vi "_Read XIC.vi"(0 "file path":path, 7 "Expt#":i32=1, 9 "MR#":i32=1, 11 "error in (no error)":errorcluster) -> (4 "Data":T6, 6 "Expt# Out":i32=1, 8 "MR# Out":i32=1, 10 "Version":i32, 15 "error out":errorcluster)   [LabVIEW 2012]
uses:
  Type/_Data.ctl
  Type/_XML Expt.ctl
  Type/_XML Lens.ctl
  Type/_Mass Range Property.ctl
  Type/_Mass Range Parameters.ctl
  Type/_RT Res Type.ctl
  Type/_GUI Method.ctl
  Type/_Lens Property.ctl
  Type/_Run Mode.ctl
panel:
  out "Steps":i32[][](array[numeric])
  in  "AcqMethod":T1[](array[typedef]) {"ScanType" format="%#.6g"; "Mass Range"."Res" items=["High/High", "Medium/Medium", "Low/Low", "High/Medium", "High/Low", "Medium/High", "Medium/Low", "Low/High", "Low/Medium"]}
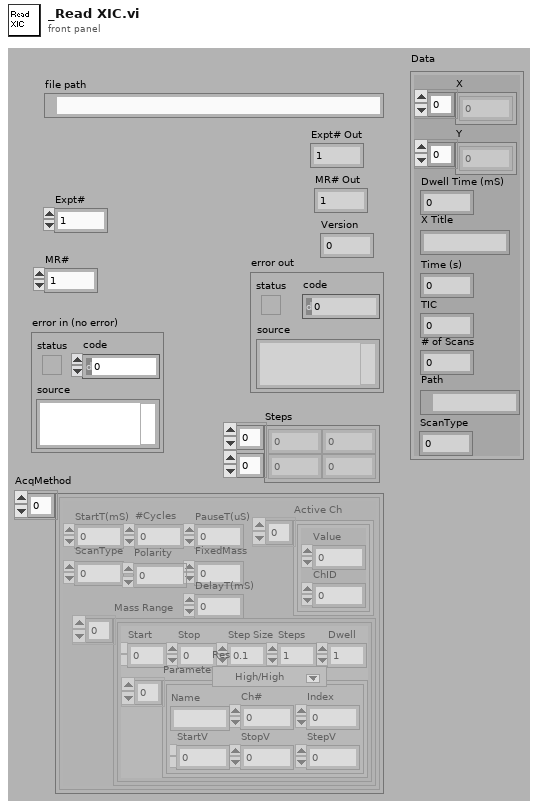
[diagram p1: front panel]
types:
  T1 = typedef "_XML Expt.ctl" = cluster{"StartT(mS)":i32, "#Cycles":i32, "PauseT(uS)":i32, "ScanType":i32, "Polarity":u8, "FixedMass":dbl, "DelayT(mS)":i32, "Active Ch":T2[], "Mass Range":T3[]}
  T2 = typedef "_XML Lens.ctl" = cluster{"Value":dbl, "ChID":u8}
  T3 = typedef "_Mass Range Property.ctl" = cluster{"Start":dbl, "Stop":dbl, "Step Size":dbl, "Steps":i32, "Dwell":dbl, "Parameters":T4[], "Res":T5}
  T4 = typedef "_Mass Range Parameters.ctl" = cluster{"Name":string, "Ch#":u8, "StartV":dbl, "StopV":dbl, "StepV":dbl, "Index":u8}
  T5 = typedef "_RT Res Type.ctl" = u16
  T6 = typedef "_Data.ctl" = cluster{"X":dbl[], "Y":dbl[], "Dwell Time (mS)":dbl, "X Title":string, "Time (s)":dbl, "TIC":u32, "# of Scans":i32, "Path":path, "ScanType":i32}
  T7 = typedef "_GUI Method.ctl" = cluster{"Lenses":T8[], "Mass Ranges":T3[], "Acquire":bool, "MCA":bool, "Q1DC EN":bool, "Q1 POL":bool, "Q3 POL":bool, "Q1 RF  EN":bool, "Averaging":bool, "Log Scale":bool, "CPS":bool, "Unit":bool, "Data Path":path, "Run Mode":T9, "Fixed Mass (amu)":dbl, "Q3DC EN":bool, "Q3 RF  EN":bool, "Negative":bool}
  T8 = typedef "_Lens Property.ctl" = cluster{"Scan Type":u8, "Scans":i32, "Time 1":dbl, "Time 2":dbl, "Value 1":dbl, "Value 2":dbl, "Step Size":dbl}
  T9 = typedef "_Run Mode.ctl" = enum16{"MRM (Q1/Q2)", "Q1 Scan", "Q1 SRM", "Q2 Scan", "Q2 SRM", "Product Scan", "Precursor Scan", "Neutral Loss", "Neutral Gain"}
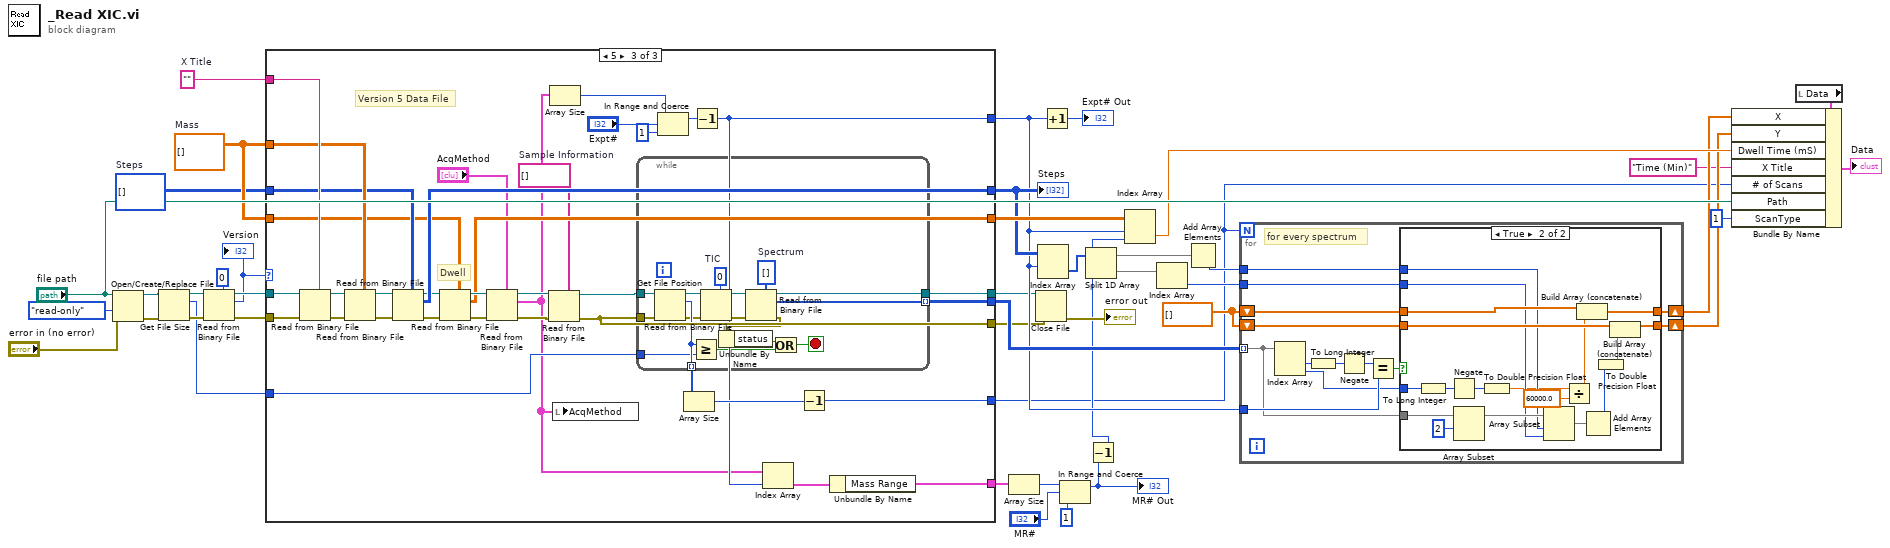
[diagram p0: block diagram]
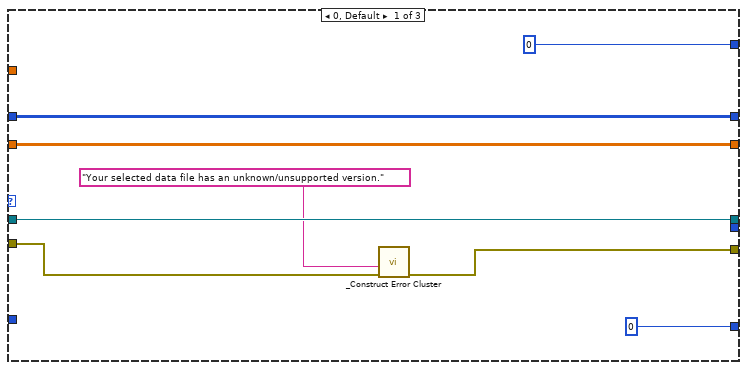
[diagram p3: hidden frame]
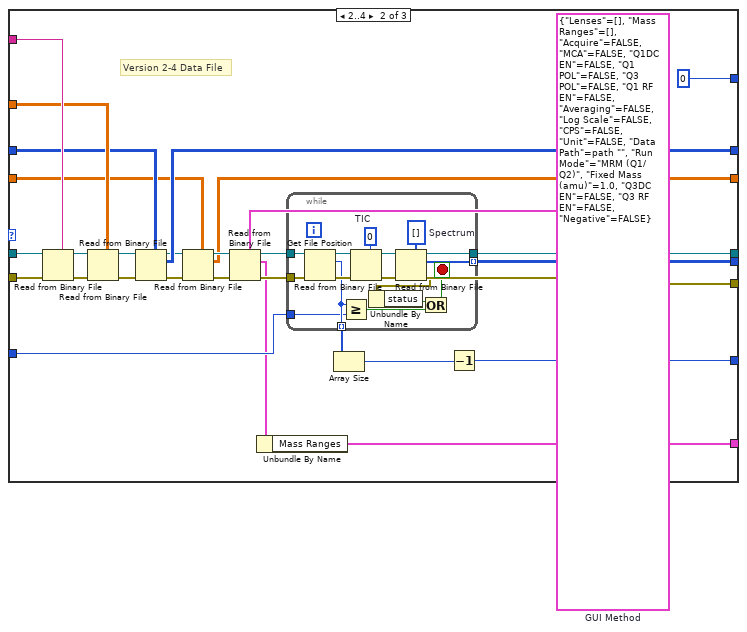
[diagram p4: hidden frame]
diagram:
  w11 = dbl[] [] ("subarray")
  w25 = ""  # X Title
  w26 = i32[][] []  # Steps
  w27 = dbl[][] []  # Mass
  n1 = Open/Create/Replace File(file path (use dialog)="file path", error in="error in (no error)", access (0:read/write)=enum16{"read/write", "read-only", "write-only"}."read-only") -> (refnum out=w38:refnum<file>, error out=w37:errorcluster)  [unwired: 4 out]
  n2 = Get File Size ("EOF")(file=w38, error in=w37) -> (refnum out=w34:refnum<file>, size (in bytes)=w30:i64, 0:w33:errorcluster)
  n3 = Read from Binary File(5:0 ("pos offset (0)"), 8:w33, 11:w34) -> (0:w31:errorcluster, 2:w24:i32, 3:w32:refnum<file>)  [unwired: 4 out]
  "Version" <- w24
  n4 = case shown="5" w24 {
    tunnel: w31 -> [w50 w77 w129]
    tunnel: w32 -> [w51 w76 w128]
    tunnel: [0 w58 w112] -> w1
    tunnel: [w51 w62 w115] -> w8
    tunnel: [w48 w61 w108] -> w7
    tunnel: w30 -> [_ w57 w111]
    tunnel: [w45 w73 w125] -> w18
    tunnel: w25 -> [_ w72 w124]
    tunnel: w27 -> [_ w71 w123]
    tunnel: w26 -> [w45 w70 w122]
    tunnel: w27 -> [w46 w64 w117]
    tunnel: [w46 w63 w116] -> w29
    tunnel: [0 ("lower limit") 0 ("lower limit") w100] -> w12
    tunnel: [_ w53 w97] -> w22
    tunnel: [_ w52 w96] -> w13
    frame 0, Default {
      n5 = call "_Construct Error Cluster.vi"("error in"=w50, "reason"="Your selected data file has an unknown/unsupported version.") -> ("error out"=w48:errorcluster)  [unwired: 2 in, 3 out]
    }
    frame 2..4 {
      w56 = T7 {"Lenses"=[], "Mass Ranges"=[], "Acquire"=FALSE, "MCA"=FALSE, "Q1DC EN"=FALSE, "Q1 POL"=FALSE, "Q3 POL"=FALSE, "Q1 RF  EN"=FALSE, "Averaging"=FALSE, "Log Scale"=FALSE, "CPS"=FALSE, "Unit"=FALSE, "Data Path"=path "", "Run Mode"=enum."MRM (Q1/Q2)", "Fixed Mass (amu)"=1.0, "Q3DC EN"=FALSE, "Q3 RF  EN"=FALSE, "Negative"=FALSE}  # GUI Method
      # "Version 2-4 Data File"
      n6 = Read from Binary File(5:w72, 8:w77, 11:w76) -> (0:w79:errorcluster, 3:w75:refnum<file>)  [unwired: 5 out]
      n7 = Read from Binary File(5:w71, 8:w79, 11:w75) -> (0:w78:errorcluster, 3:w74:refnum<file>)  [unwired: 5 out]
      n8 = Read from Binary File(5:w70, 8:w78, 11:w74) -> (0:w66:errorcluster, 2:w73:i32[][], 3:w67:refnum<file>)  [unwired: 4 out]
      n9 = Read from Binary File(5:w64, 8:w66, 11:w67) -> (0:w68:errorcluster, 2:w63:dbl[][], 3:w65:refnum<file>)  [unwired: 4 out]
      n10 = Read from Binary File(5:w56, 8:w68, 11:w65) -> (0:w61:errorcluster, 2:w54:T7, 3:w69:refnum<file>)  [unwired: 4 out]
      n11 = Unbundle By Name(w54) -> ("Mass Ranges"=w53:T3[])
      n12 = while {
        tunnel: w69 -> [w95]
        tunnel: w61 -> [w94]
        tunnel: [w92] -> w62
        tunnel: [w91] -> w60 mode=indexing
        tunnel: w57 -> [w90]
        tunnel: [w80] -> w52 mode=indexing
        stop <- w87 stop-if-true
        w82 = u32 0  # TIC
        w93 = u32[] []  # Spectrum
        n13 = Get File Position(4:w94, 7:w95) -> (0:w83:errorcluster, 2:w91:i64, 3:w85:refnum<file>)
        n14 = Greater Or Equal?(x=w91, y=w90) -> (x >= y?=w88:bool)
        n15 = Read from Binary File(5:w82, 8:w83, 11:w85) -> (0:w86:errorcluster, 3:w84:refnum<file>)  [unwired: 5 out]
        n16 = Read from Binary File(5:w93, 8:w86, 11:w84) -> (0:w81:errorcluster, 2:w80:u32[], 3:w92:refnum<file>)  [unwired: 4 out]
        n17 = Unbundle By Name(w81) -> ("status"=w89:bool)
        n18 = Or(x=w89, y=w88) -> (x .or. y?=w87:bool)
      }
      n19 = Array Size(array=w60) -> (size(s)=w59:i32)
      n20 = Decrement(x=w59) -> (x-1=w58:i32)
    }
    frame 5 {
      w106 = string[] []  # Sample Information
      # "Dwell"
      # "Version 5 Data File"
      n21 = Read from Binary File(5:w124, 8:w129, 11:w128) -> (0:w131:errorcluster, 3:w127:refnum<file>)  [unwired: 5 out]
      n22 = Read from Binary File(5:w123, 8:w131, 11:w127) -> (0:w130:errorcluster, 3:w126:refnum<file>)  [unwired: 5 out]
      n23 = Read from Binary File(5:w122, 8:w130, 11:w126) -> (0:w119:errorcluster, 2:w125:i32[][], 3:w120:refnum<file>)  [unwired: 4 out]
      n24 = Read from Binary File(5:w117, 8:w119, 11:w120) -> (0:w121:errorcluster, 2:w116:dbl[][], 3:w118:refnum<file>)  [unwired: 4 out]
      n25 = Read from Binary File(5:"AcqMethod", 8:w121, 11:w118) -> (0:w107:errorcluster, 2:w98:T1[], 3:w110:refnum<file>)  [unwired: 4 out]
      n26 = Read from Binary File(5:w106, 8:w107, 11:w110) -> (0:w108:errorcluster, 3:w109:refnum<file>)  [unwired: 5 out]
      n27 = Array Size(array=w98) -> (size(s)=w101:i32)
      n28 = local write "AcqMethod"(w98) -> ()
      n29 = while {
        tunnel: w109 -> [w147]
        tunnel: w108 -> [w146]
        tunnel: [w144] -> w115
        tunnel: [w143] -> w114 mode=indexing
        tunnel: w111 -> [w142]
        tunnel: [w132] -> w96 mode=indexing
        stop <- w139 stop-if-true
        w134 = u32 0  # TIC
        w145 = u32[] []  # Spectrum
        n30 = Get File Position(4:w146, 7:w147) -> (0:w135:errorcluster, 2:w143:i64, 3:w137:refnum<file>)
        n31 = Greater Or Equal?(x=w143, y=w142) -> (x >= y?=w140:bool)
        n32 = Read from Binary File(5:w134, 8:w135, 11:w137) -> (0:w138:errorcluster, 3:w136:refnum<file>)  [unwired: 5 out]
        n33 = Read from Binary File(5:w145, 8:w138, 11:w136) -> (0:w133:errorcluster, 2:w132:u32[], 3:w144:refnum<file>)  [unwired: 4 out]
        n34 = Unbundle By Name(w133) -> ("status"=w141:bool)
        n35 = Or(x=w141, y=w140) -> (x .or. y?=w139:bool)
      }
      n36 = In Range and Coerce(upper limit=w101, x="Expt#", lower limit=1) -> (coerced(x)=w102:i32)  [unwired: 1 out]
      n37 = Array Size(array=w114) -> (size(s)=w113:i32)
      n38 = Decrement(x=w102) -> (x-1=w100:i32)
      n39 = Index Array(array=w98, index=w100) -> (element=w99:T1)
      n40 = Decrement(x=w113) -> (x-1=w112:i32)
      n41 = Unbundle By Name(w99) -> ("Mass Range"=w97:T3[])
    }
  }
  "Steps" <- w18
  n42 = Array Size(array=w22) -> (size(s)=w20:i32)
  n43 = Close File(refnum=w8, error in=w7) -> (error out=→"error out":errorcluster)  [unwired: 1 out]
  n44 = Index Array(array=w18, index (row)=w12) -> (element=w17:i32[])  [unwired: 1 in]
  n45 = Increment(x=w12) -> (x+1=→"Expt# Out":i32)
  n46 = In Range and Coerce(upper limit=w20, x="MR#", lower limit=1) -> (coerced(x)=w16:i32)  [unwired: 1 out]
  "MR# Out" <- w16
  n47 = Decrement(x=w16) -> (x-1=w6:i32)
  n48 = Split 1D Array(array=w17, index=w6) -> (first subarray=w15:i32[], second subarray=w14:i32[])
  n49 = Index Array(array=w29, index (row)=w12, index (col)=w6) -> (element=w28:dbl)
  n50 = Index Array(array=w14) -> (element=w9:i32)  [unwired: 1 in]
  n51 = Add Array Elements(numeric array=w15) -> (sum=w10:i32)
  n52 = for {
    N: w1 -> [_]
    tunnel: w13 -> [w150] mode=indexing
    shift-right: [w153] -> w5
    shift-left: w11 -> [w155]
    shift-right: [w152] -> w4
    shift-left: w11 -> [w154]
    tunnel: w12 -> [w157]
    tunnel: w10 -> [w149]
    tunnel: w9 -> [w148]
    # "for every spectrum"
    n53 = Index Array(array=w150) -> (element #1=w159:u32, element #2=w151:u32)  [unwired: 2 in]
    n54 = To Long Integer(number=w159) -> (32bit integer=w160:i32)
    n55 = Negate(x=w160) -> (-x=w158:i32)
    n56 = Equal?(x=w158, y=w157) -> (x = y?=w156:bool)
    n57 = case shown="True" w156 {
      tunnel: w155 -> [w162 w178]
      tunnel: w154 -> [w161 w171]
      tunnel: [w162 w176] -> w153
      tunnel: [w161 w170] -> w152
      tunnel: w151 -> [_ w179]
      tunnel: w150 -> [_ w174]
      tunnel: w149 -> [_ w167]
      tunnel: w148 -> [_ w166]
      frame False {
      }
      frame True {
        n58 = To Long Integer(number=w179) -> (32bit integer=w180:i32)
        n59 = Negate(x=w180) -> (-x=w177:i32)
        n60 = Array Subset(array=w174, index=2) -> (w173:u32[])  [unwired: 1 in]
        n61 = To Double Precision Float(number=w177) -> (double precision float=w164:dbl)
        n62 = Array Subset(array=w173, index=w167, length=w166) -> (w172:u32[])
        n63 = Divide(x=w164, y=60000.0) -> (x/y=w163:dbl)
        n64 = Build Array (concatenate)(w178, w163) -> (w176:dbl[])
        n65 = Add Array Elements(numeric array=w172) -> (sum=w168:u32)
        n66 = To Double Precision Float(number=w168) -> (double precision float=w169:dbl)
        n67 = Build Array (concatenate)(w171, w169) -> (w170:dbl[])
      }
    }
  }
  n68 = local read "Data"() -> (w41:T6)
  n69 = Bundle By Name(cluster=w41, "X"=w5, "Y"=w4, "Dwell Time (mS)"=w28, "X Title"="Time (Min)", "# of Scans"=w1, "Path"="file path", "ScanType"=1) -> (→"Data":T6)
